vi "Enqueue-Process1-action.vi"(8 "error in (no error)":errorcluster, 9 "Timeout (ms)":i32=-1, 10 "Action":T1, 11 "State queue in":T2) -> (0 "error out":errorcluster, 1 "Timed out?":bool, 3 "State queue out":T2)   [LabVIEW 2013, in "MaterialCharacterization.lvlib" / "MC-Main.lvclass"]
doc: "Use this template to build a VI to use as a subVI."
uses:
  MC-Main.lvclass
  Object-reference.ctl
  Process1-actions.ctl
  MC-Main.lvclass/MC-Main.ctl
  Read Process 1 queue.vi
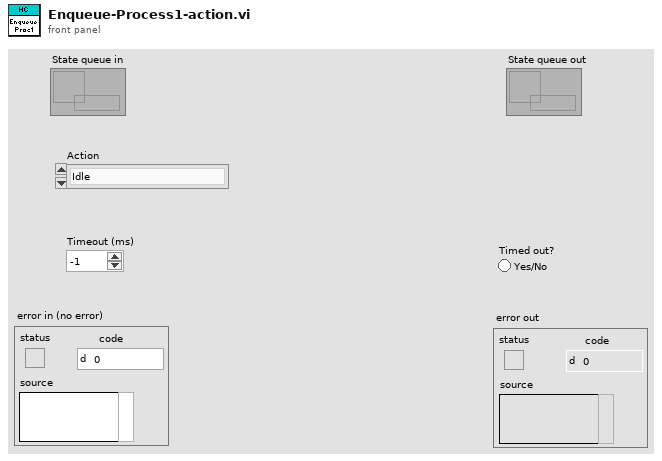
[diagram p1: front panel]
types:
  T1 = typedef "MaterialCharacterization.lvlib/MC-Main.lvclass/Process1-actions.ctl" = enum16{"Idle", "Activate", "Analyse scan file", "Convert SM1000positions", "Measure SM1000 timings", "Measure laser timings", "Stop", "Abort", "Exit"}
  T2 = typedef "MaterialCharacterization.lvlib/MC-Main.lvclass/Object-reference.ctl" = refnum<data-value>
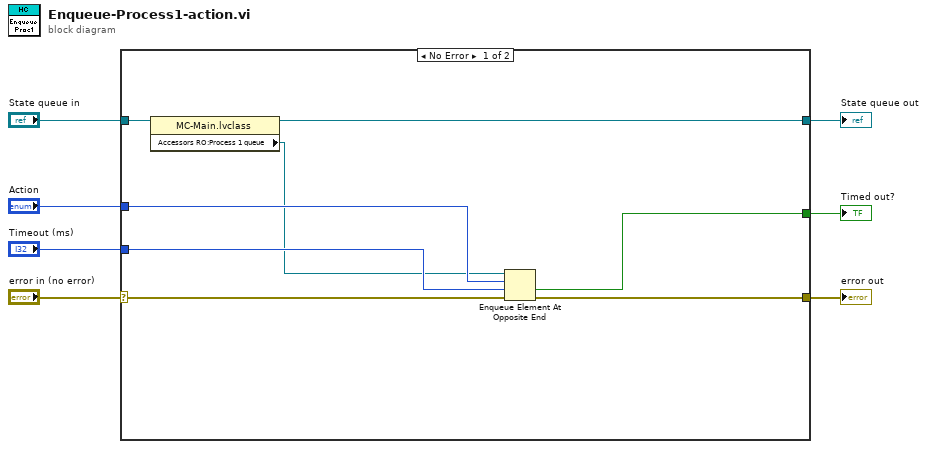
[diagram p0: block diagram]
diagram:
  n1 = case shown="No Error" "error in (no error)" {
    selector: "error in (no error)" -> [w8 w17]
    tunnel: [w14 w17] -> w6
    tunnel: "Action" -> [w13 _]
    tunnel: "State queue in" -> [w15 w16]
    tunnel: [w9 w16] -> w4
    tunnel: "Timeout (ms)" -> [w12 _]
    tunnel: [w11 _] -> w2
    frame No Error {
      n2 = property class="MC-Main.lvclass"(reference=w15) -> (reference out=w9:T2, "Accessors RO:Process 1 queue"=w10:refnum<queue>)  [unwired: 1 in, 1 out]
      n3 = Enqueue Element At Opposite End(queue=w10, element=w13, timeout in ms (-1)=w12, error in (no error)=w8) -> (timed out?=w11:bool, error out=w14:errorcluster)  [unwired: 1 out]
    }
    frame Error {
    }
  }
  "error out" <- w6
  "State queue out" <- w4
  "Timed out?" <- w2
